vi "Version_2.0_Single_Column_Code.vi"() -> ()   [LabVIEW 2020] (continued)
                        n8405 = local write "Reminder of the \nVolume to be \nPumped"(w8823) -> ()
                      }
                      frame #1 {
                        n8406 = stacked-sequence {
                          frame #0 {
                            # "Switch to Port-4"
                            # "Port-4 of pump is connected to Buffer-A"
                            n8407 = local read "VISA Refnum in\nfor Pump"() -> (w8907:refnum<visa-resource-name>)
                            n8408 = local read "Port for \nA2-Wash"() -> (w8906:string)
                            n8409 = call "PortChanger (SubVI).vi"("Port Number"=w8906, "VISA Refnum in"=w8907) -> ()  [unwired: 10 in]
                          }
                          frame #1 {
                            n8410 = local read "VISA Refnum in\nfor Pump"() -> (w8908:refnum<visa-resource-name>)
                            n8411 = call "ProcessCompletionWaiter (SubVI).vi"("VISA Refnum in"=w8908) -> ()  [unwired: 11 in]
                          }
                          frame #2 {
                            n8412 = local read "Buffer-A2 PickUp \nFlow Rate (ul/min)"() -> (w8911:dbl)
                            n8413 = local read "Buffer-A2 Pumping\nResolution"() -> (w8910:T2)
                            n8414 = local read "VISA Refnum in\nfor Pump"() -> (w8913:refnum<visa-resource-name>)
                            n8415 = local read "Reminder of the \nVolume to be \nPumped"() -> (w8909:dbl)
                            n8416 = local read "Volume of Syringe"() -> (w8912:dbl)
                            n8417 = call "RPickUp(SubVI).vi"("Volume to be picked up"=w8909, "Volume of Syringe"=w8912, "Resolution of PickUP"=w8910, "PickUp Flow Rate (ul/min)"=w8911, "VISA Refnum in"=w8913) -> ()  [unwired: 6 in, 1 out]
                          }
                          frame #3 {
                            n8418 = local read "Stopper that ends \nthe main loops"() -> (w8914:bool)
                            n8419 = local read "VISA Refnum in\nfor Pump"() -> (w8915:refnum<visa-resource-name>)
                            n8420 = case shown="True" w8914 {
                              frame False {
                              }
                              frame True {
                                n8421 = local read "VISA Refnum in\nfor Pump"() -> (w8916:refnum<visa-resource-name>)
                                n8422 = call "HardStopCurrentProcess (SubVI).vi"("VISA Refnum in"=w8916) -> ()  [unwired: 11 in]
                              }
                            }
                            n8423 = call "ProcessCompletionWaiter (SubVI).vi"("VISA Refnum in"=w8915) -> ()  [unwired: 11 in]
                          }
                          frame #4 {
                            # "Reads the initial Plunger Position for computing the volume dispensed"
                            n8424 = local read "VISA Refnum in\nfor Pump"() -> (w8918:refnum<visa-resource-name>)
                            n8425 = call "AbsolutePlungerPosition (SubVI).vi"("VISA Refnum in"=w8918) -> ("Plunger Position"=w8917:i32)  [unwired: 10 in]
                            n8426 = local write "Initial Plunger Position"(w8917) -> ()
                          }
                          frame #5 {
                            # "Switch to Port-2"
                            # "Port-2 of the pump is conncted to column-1 of chip"
                            n8427 = local read "VISA Refnum in\nfor Pump"() -> (w8920:refnum<visa-resource-name>)
                            n8428 = call "PortChanger (SubVI).vi"("Port Number"="2", "VISA Refnum in"=w8920) -> ()  [unwired: 10 in]
                          }
                          frame #6 {
                            n8429 = local read "Stopper that ends \nthe main loops"() -> (w8921:bool)
                            n8430 = local read "VISA Refnum in\nfor Pump"() -> (w8922:refnum<visa-resource-name>)
                            n8431 = case shown="True" w8921 {
                              frame False {
                              }
                              frame True {
                                n8432 = local read "VISA Refnum in\nfor Pump"() -> (w8923:refnum<visa-resource-name>)
                                n8433 = call "HardStopCurrentProcess (SubVI).vi"("VISA Refnum in"=w8923) -> ()  [unwired: 11 in]
                              }
                            }
                            n8434 = call "ProcessCompletionWaiter (SubVI).vi"("VISA Refnum in"=w8922) -> ()  [unwired: 11 in]
                          }
                          frame #7 {
                            # "Keeps the AMF valve after column-1 open and valve after column-2 closed"
                            n8435 = local read "Buffer-A2 Dispense\nFlow Rate (ul/min)"() -> (w8936:dbl)
                            n8436 = local read "Buffer-A2 Pumping\nResolution"() -> (w8935:T2)
                            n8437 = local read "VISA Refnum in\nfor Pump"() -> (w8938:refnum<visa-resource-name>)
                            n8438 = local write "Pause Data Collection"(FALSE ("Pause Data Collection")) -> ()
                            n8439 = local write "Valve V3 Open"(TRUE ("Valve V3 Open")) -> ()
                            n8440 = local write "Valve V4 Open"(TRUE ("Valve V4 Open")) -> ()
                            n8441 = local write "Valve V1 Open"(TRUE ("Valve V1 Open")) -> ()
                            n8442 = local write "Valve V2 Open"(FALSE ("Valve V2 Open")) -> ()
                            n8443 = local read "Volume of Syringe"() -> (w8937:dbl)
                            n8444 = call "GoToAbsolutePosition(SubVI).vi"("Absolute Volume Position in Syringe (in ul)"=0.0 ("Volume to be Dispensed"), "Volume of Syringe"=w8937, "Resolution of Pumping"=w8935, "Flow Rate (ul/min)"=w8936, "VISA Refnum in"=w8938) -> ()  [unwired: 6 in, 1 out]
                            n8445 = local write "External Valve \nOpen"(FALSE ("External Valve \nOpen")) -> ()
                            n8446 = local write "Valve V5 Open"(TRUE ("Valve V5 Open")) -> ()
                            n8447 = local write "Valve V8 Open"(TRUE ("Valve V8 Open")) -> ()
                            n8448 = local write "Valve V6 Open"(TRUE ("Valve V6 Open")) -> ()
                            n8449 = local write "Valve V7 Open"(TRUE ("Valve V7 Open")) -> ()
                          }
                          frame #8 {
                            n8450 = local read "Initial Plunger Position"() -> (w8941:dbl)
                            n8451 = local read "Buffer-A2 Pumping\nResolution"() -> (w8940:T2)
                            n8452 = local read "VISA Refnum in\nfor Pump"() -> (w8942:refnum<visa-resource-name>)
                            n8453 = local read "Volume of Syringe"() -> (w8939:dbl)
                            n8454 = while {
                              tunnel: w8941 -> [w8948]
                              tunnel: w8942 -> [w8947]
                              tunnel: w8940 -> [w8946]
                              tunnel: w8939 -> [w8945]
                              stop <- w8943 stop-if-true
                              n8455 = Wait (ms)(milliseconds to wait=u32 100) -> ()  [unwired: 1 out]
                              n8456 = stacked-sequence {
                                tunnel: w8948 -> [w8954 _]
                                tunnel: w8947 -> [w8953 w8974]
                                tunnel: w8946 -> [w8952 _]
                                tunnel: w8945 -> [w8951 _]
                                tunnel: [_ w8971] -> w8943
                                frame #0 {
                                n8457 = call "AbsolutePlungerPosition (SubVI).vi"("VISA Refnum in"=w8953) -> ("Plunger Position"=w8950:i32)  [unwired: 10 in]
                                n8458 = case shown="\"Standard Pumping\", Default" w8952 {
                                tunnel: w8954 -> [w8959 w8968]
                                tunnel: w8950 -> [w8960 w8967]
                                tunnel: [w8958 w8965] -> w8949
                                tunnel: w8951 -> [w8957 w8966]
                                frame "Standard Pumping", Default {
                                n8459 = Subtract(x=w8959, y=w8960) -> (x-y=w8956:dbl)
                                n8460 = Absolute Value(x=w8956) -> (abs(x)=w8955:dbl)
                                n8461 = Multiply(x=w8955, y=w8957) -> (x*y=w8962:dbl)
                                n8462 = Divide(x=w8962, y=3000.0) -> (x/y=w8958:dbl)
                                }
                                frame "High Resolution Pumping" {
                                n8463 = Subtract(x=w8968, y=w8967) -> (x-y=w8964:dbl)
                                n8464 = Absolute Value(x=w8964) -> (abs(x)=w8963:dbl)
                                n8465 = Multiply(x=w8963, y=w8966) -> (x*y=w8970:dbl)
                                n8466 = Divide(x=w8970, y=24000.0) -> (x/y=w8965:dbl)
                                }
                                }
                                n8467 = local write "Volume being Injected \nin this process"(w8949) -> ()
                                }
                                frame #1 {
                                n8468 = local read "Stop for End of \nExperiment \nand Data Writing"() -> (w8973:bool)
                                n8469 = call "LSPOneStatus (SubVI).vi"("VISA Refnum in"=w8974) -> ("read buffer"=w8976:string)  [unwired: 10 in]
                                n8470 = call <vilib>:"Trim Whitespace.vi"("string"=w8976) -> ("trimmed string"=w8975:string)  [unwired: 1 in]
                                n8471 = Equal?(x=w8975, y="/0`\u0003") -> (x = y?=w8972:bool)
                                n8472 = Or(x=w8972, y=w8973) -> (x .or. y?=w8971:bool)
                                }
                              }
                            }
                          }
                          frame #9 {
                            n8473 = local read "Stop for End of \nExperiment \nand Data Writing"() -> (w8978:bool)
                            n8474 = local write "Pause Data Collection"(TRUE ("Pause Data Collection")) -> ()
                            n8475 = local write "Valve V2 Open"(FALSE ("Valve V2 Open")) -> ()
                            n8476 = local write "Start the Process"(FALSE) -> ()
                            n8477 = local write "Valve V1 Open"(FALSE ("Valve V1 Open")) -> ()
                            n8478 = case shown="True" w8978 {
                              frame False {
                              }
                              frame True {
                                n8479 = local read "VISA Refnum in\nfor Pump"() -> (w8984:refnum<visa-resource-name>)
                                n8480 = call "HardStopCurrentProcess (SubVI).vi"("VISA Refnum in"=w8984) -> ()  [unwired: 11 in]
                              }
                            }
                            n8481 = Wait (ms)(milliseconds to wait=u32 500) -> ()  [unwired: 1 out]
                          }
                          frame #10 {
                            n8482 = local write "Volume being Injected \nin this process"(0.0 ("Volume being Injected \nin this process")) -> ()
                          }
                        }
                      }
                    }
                  }
                }
              }
              frame True {
                n8483 = local write "Pause Data Collection"(FALSE ("Pause Data Collection")) -> ()
              }
            }
          }
          frame "Inject Buffer B, Column 1 with 4 SOD Valves" {
            n8484 = local read "Stopper that ends \nthe main loops"() -> (w8987:bool)
            n8485 = case shown="False" w8987 {
              frame False {
                n8486 = local read "Start the Process"() -> (w8988:bool)
                n8487 = case shown="True" w8988 {
                  frame False {
                    n8488 = local read "Stopper that ends \nthe main loops"() -> (w8990:bool)
                    n8489 = local read "Start the Process"() -> (w8989:bool)
                    n8490 = Or(x=w8990, y=w8989) -> (x .or. y?=w8991:bool)
                    n8491 = case shown="False" w8991 {
                      frame False {
                        n8492 = while {
                          stop <- w8994 stop-if-true
                          n8493 = local read "Stop for End of \nExperiment \nand Data Writing"() -> (w8993:bool)
                          n8494 = local read "Stopper that ends \nthe main loops"() -> (w8996:bool)
                          n8495 = local read "Start the Process"() -> (w8995:bool)
                          n8496 = Wait (ms)(milliseconds to wait=u32 10) -> ()  [unwired: 1 out]
                          n8497 = Or(x=w8996, y=w8995) -> (x .or. y?=w8994:bool)
                          n8498 = local write "Stopper that ends \nthe main loops"(w8993) -> ()
                        }
                        n8499 = One Button Dialog(message="Please Select the Process and Press 'Start the Process' Button") -> ()  [unwired: 1 in, 1 out]
                      }
                      frame True {
                      }
                    }
                  }
                  frame True {
                    n8500 = stacked-sequence {
                      frame #0 {
                        n8501 = local read "Apparent Volume\nof Syringe"() -> (w9000:dbl)
                        n8502 = local read "Buffer-B Volume \nto be  Pumped"() -> (w9001:dbl)
                        n8503 = Quotient & Remainder(x=w9001, y=w9000) -> (x-y*floor(x/y)=w8998:dbl, floor(x/y)=w8999:dbl)
                        n8504 = for {
                          N: w8999 -> [_]
                          n8505 = stacked-sequence {
                            frame #0 {
                              # "Switch to Port-7"
                              # "Port-7 of pump is connected to Buffer-B"
                              n8506 = local read "VISA Refnum in\nfor Pump"() -> (w9003:refnum<visa-resource-name>)
                              n8507 = local read "Port for \nB-Elution"() -> (w9002:string)
                              n8508 = call "PortChanger (SubVI).vi"("Port Number"=w9002, "VISA Refnum in"=w9003) -> ()  [unwired: 10 in]
                            }
                            frame #1 {
                              n8509 = local read "VISA Refnum in\nfor Pump"() -> (w9004:refnum<visa-resource-name>)
                              n8510 = call "ProcessCompletionWaiter (SubVI).vi"("VISA Refnum in"=w9004) -> ()  [unwired: 11 in]
                            }
                            frame #2 {
                              n8511 = local read "Buffer-B PickUp \nFlow Rate (ul/min)"() -> (w9007:dbl)
                              n8512 = local read "Buffer-B Pumping\nResolution"() -> (w9006:T2)
                              n8513 = local read "VISA Refnum in\nfor Pump"() -> (w9009:refnum<visa-resource-name>)
                              n8514 = local read "Apparent Volume\nof Syringe"() -> (w9005:dbl)
                              n8515 = local read "Volume of Syringe"() -> (w9008:dbl)
                              n8516 = call "RPickUp(SubVI).vi"("Volume to be picked up"=w9005, "Volume of Syringe"=w9008, "Resolution of PickUP"=w9006, "PickUp Flow Rate (ul/min)"=w9007, "VISA Refnum in"=w9009) -> ()  [unwired: 6 in, 1 out]
                            }
                            frame #3 {
                              n8517 = local read "Stopper that ends \nthe main loops"() -> (w9010:bool)
                              n8518 = local read "VISA Refnum in\nfor Pump"() -> (w9011:refnum<visa-resource-name>)
                              n8519 = case shown="True" w9010 {
                                frame False {
                                }
                                frame True {
                                n8520 = local read "VISA Refnum in\nfor Pump"() -> (w9012:refnum<visa-resource-name>)
                                n8521 = call "HardStopCurrentProcess (SubVI).vi"("VISA Refnum in"=w9012) -> ()  [unwired: 11 in]
                                }
                              }
                              n8522 = call "ProcessCompletionWaiter (SubVI).vi"("VISA Refnum in"=w9011) -> ()  [unwired: 11 in]
                            }
                            frame #4 {
                              # "Reads the initial Plunger Position for computing the volume dispensed"
                              n8523 = local read "VISA Refnum in\nfor Pump"() -> (w9014:refnum<visa-resource-name>)
                              n8524 = call "AbsolutePlungerPosition (SubVI).vi"("VISA Refnum in"=w9014) -> ("Plunger Position"=w9013:i32)  [unwired: 10 in]
                              n8525 = local write "Initial Plunger Position"(w9013) -> ()
                            }
                            frame #5 {
                              # "Switch to Port-8"
                              # "Port-8 of the pump is conncted to column-1 of chip"
                              n8526 = local read "VISA Refnum in\nfor Pump"() -> (w9016:refnum<visa-resource-name>)
                              n8527 = call "PortChanger (SubVI).vi"("Port Number"="8", "VISA Refnum in"=w9016) -> ()  [unwired: 10 in]
                            }
                            frame #6 {
                              n8528 = local read "Stopper that ends \nthe main loops"() -> (w9017:bool)
                              n8529 = local read "VISA Refnum in\nfor Pump"() -> (w9018:refnum<visa-resource-name>)
                              n8530 = case shown="True" w9017 {
                                frame False {
                                }
                                frame True {
                                n8531 = local read "VISA Refnum in\nfor Pump"() -> (w9019:refnum<visa-resource-name>)
                                n8532 = call "HardStopCurrentProcess (SubVI).vi"("VISA Refnum in"=w9019) -> ()  [unwired: 11 in]
                                }
                              }
                              n8533 = call "ProcessCompletionWaiter (SubVI).vi"("VISA Refnum in"=w9018) -> ()  [unwired: 11 in]
                            }
                            frame #7 {
                              # "Keeps the AMF valve after column-1 open and valve after column-2 closed"
                              n8534 = local read "Buffer-B Dispense\nFlow Rate (ul/min)"() -> (w9032:dbl)
                              n8535 = local read "Buffer-B Pumping\nResolution"() -> (w9031:T2)
                              n8536 = local read "VISA Refnum in\nfor Pump"() -> (w9034:refnum<visa-resource-name>)
                              n8537 = local write "Pause Data Collection"(FALSE ("Pause Data Collection")) -> ()
                              n8538 = local write "Valve V1 Open"(TRUE ("Valve V1 Open")) -> ()
                              n8539 = local write "Valve V3 Open"(FALSE ("Valve V3 Open")) -> ()
                              n8540 = local write "Valve V2 Open"(TRUE ("Valve V2 Open")) -> ()
                              n8541 = local write "Valve V4 Open"(FALSE ("Valve V4 Open")) -> ()
                              n8542 = local read "Volume of Syringe"() -> (w9033:dbl)
                              n8543 = call "GoToAbsolutePosition(SubVI).vi"("Absolute Volume Position in Syringe (in ul)"=0.0 ("Volume to be Dispensed"), "Volume of Syringe"=w9033, "Resolution of Pumping"=w9031, "Flow Rate (ul/min)"=w9032, "VISA Refnum in"=w9034) -> ()  [unwired: 6 in, 1 out]
                              n8544 = local write "External Valve \nOpen"(TRUE ("External Valve \nOpen")) -> ()
                              n8545 = local write "Valve V8 Open"(FALSE ("Valve V8 Open")) -> ()
                              n8546 = local write "Valve V6 Open"(FALSE ("Valve V6 Open")) -> ()
                              n8547 = local write "Valve V7 Open"(FALSE ("Valve V7 Open")) -> ()
                              n8548 = local write "Valve V5 Open"(FALSE ("Valve V5 Open")) -> ()
                            }
                            frame #8 {
                              n8549 = local read "Initial Plunger Position"() -> (w9037:dbl)
                              n8550 = local read "Buffer-B Pumping\nResolution"() -> (w9036:T2)
                              n8551 = local read "VISA Refnum in\nfor Pump"() -> (w9038:refnum<visa-resource-name>)
                              n8552 = local read "Volume of Syringe"() -> (w9035:dbl)
                              n8553 = while {
                                tunnel: w9037 -> [w9044]
                                tunnel: w9038 -> [w9043]
                                tunnel: w9036 -> [w9042]
                                tunnel: w9035 -> [w9041]
                                stop <- w9039 stop-if-true
                                n8554 = Wait (ms)(milliseconds to wait=u32 100) -> ()  [unwired: 1 out]
                                n8555 = stacked-sequence {
                                tunnel: w9044 -> [w9050 _]
                                tunnel: w9043 -> [w9049 w9070]
                                tunnel: w9042 -> [w9048 _]
                                tunnel: w9041 -> [w9047 _]
                                tunnel: [_ w9067] -> w9039
                                frame #0 {
                                n8556 = call "AbsolutePlungerPosition (SubVI).vi"("VISA Refnum in"=w9049) -> ("Plunger Position"=w9046:i32)  [unwired: 10 in]
                                n8557 = case shown="\"Standard Pumping\", Default" w9048 {
                                tunnel: w9050 -> [w9055 w9064]
                                tunnel: w9046 -> [w9056 w9063]
                                tunnel: [w9054 w9061] -> w9045
                                tunnel: w9047 -> [w9053 w9062]
                                frame "Standard Pumping", Default {
                                n8558 = Subtract(x=w9055, y=w9056) -> (x-y=w9052:dbl)
                                n8559 = Absolute Value(x=w9052) -> (abs(x)=w9051:dbl)
                                n8560 = Multiply(x=w9051, y=w9053) -> (x*y=w9058:dbl)
                                n8561 = Divide(x=w9058, y=3000.0) -> (x/y=w9054:dbl)
                                }
                                frame "High Resolution Pumping" {
                                n8562 = Subtract(x=w9064, y=w9063) -> (x-y=w9060:dbl)
                                n8563 = Absolute Value(x=w9060) -> (abs(x)=w9059:dbl)
                                n8564 = Multiply(x=w9059, y=w9062) -> (x*y=w9066:dbl)
                                n8565 = Divide(x=w9066, y=24000.0) -> (x/y=w9061:dbl)
                                }
                                }
                                n8566 = local write "Volume being Injected \nin this process"(w9045) -> ()
                                }
                                frame #1 {
                                n8567 = call "LSPOneStatus (SubVI).vi"("VISA Refnum in"=w9070) -> ("read buffer"=w9072:string)  [unwired: 10 in]
                                n8568 = local read "Stopper that ends \nthe main loops"() -> (w9069:bool)
                                n8569 = call <vilib>:"Trim Whitespace.vi"("string"=w9072) -> ("trimmed string"=w9071:string)  [unwired: 1 in]
                                n8570 = Equal?(x=w9071, y="/0`\u0003") -> (x = y?=w9068:bool)
                                n8571 = Or(x=w9068, y=w9069) -> (x .or. y?=w9067:bool)
                                }
                                }
                              }
                            }
                            frame #9 {
                              n8572 = local read "Stopper that ends \nthe main loops"() -> (w9074:bool)
                              n8573 = local write "Pause Data Collection"(TRUE ("Pause Data Collection")) -> ()
                              n8574 = local write "Valve V2 Open"(FALSE ("Valve V2 Open")) -> ()
                              n8575 = local write "Valve V4 Open"(FALSE ("Valve V4 Open")) -> ()
                              n8576 = Wait (ms)(milliseconds to wait=u32 500) -> ()  [unwired: 1 out]
                              n8577 = local write "Valve V1 Open"(FALSE ("Valve V1 Open")) -> ()
                              n8578 = local write "Valve V3 Open"(FALSE ("Valve V3 Open")) -> ()
                              n8579 = case shown="True" w9074 {
                                frame False {
                                }
                                frame True {
                                n8580 = local read "VISA Refnum in\nfor Pump"() -> (w9084:refnum<visa-resource-name>)
                                n8581 = call "HardStopCurrentProcess (SubVI).vi"("VISA Refnum in"=w9084) -> ()  [unwired: 11 in]
                                }
                              }
                              n8582 = local write "Valve V5 Open"(FALSE ("Valve V5 Open")) -> ()
                              n8583 = local write "Valve V6 Open"(FALSE ("Valve V6 Open")) -> ()
                              n8584 = local write "Valve V7 Open"(FALSE ("Valve V7 Open")) -> ()
                            }
                            frame #10 {
                              n8585 = local write "Volume being Injected \nin this process"(0.0 ("Volume being Injected \nin this process")) -> ()
                            }
                          }
                        }
                        n8586 = local write "Reminder of the \nVolume to be \nPumped"(w8998) -> ()
                      }
                      frame #1 {
                        n8587 = stacked-sequence {
                          frame #0 {
                            # "Switch to Port-7"
                            # "Port-7 of pump is connected to Buffer-B"
                            n8588 = local read "VISA Refnum in\nfor Pump"() -> (w9087:refnum<visa-resource-name>)
                            n8589 = local read "Port for \nB-Elution"() -> (w9086:string)
                            n8590 = call "PortChanger (SubVI).vi"("Port Number"=w9086, "VISA Refnum in"=w9087) -> ()  [unwired: 10 in]
                          }
                          frame #1 {
                            n8591 = local read "VISA Refnum in\nfor Pump"() -> (w9088:refnum<visa-resource-name>)
                            n8592 = call "ProcessCompletionWaiter (SubVI).vi"("VISA Refnum in"=w9088) -> ()  [unwired: 11 in]
                          }
                          frame #2 {
                            n8593 = local read "Buffer-B PickUp \nFlow Rate (ul/min)"() -> (w9091:dbl)
                            n8594 = local read "Buffer-B Pumping\nResolution"() -> (w9090:T2)
                            n8595 = local read "VISA Refnum in\nfor Pump"() -> (w9093:refnum<visa-resource-name>)
                            n8596 = local read "Reminder of the \nVolume to be \nPumped"() -> (w9089:dbl)
                            n8597 = local read "Volume of Syringe"() -> (w9092:dbl)
                            n8598 = call "RPickUp(SubVI).vi"("Volume to be picked up"=w9089, "Volume of Syringe"=w9092, "Resolution of PickUP"=w9090, "PickUp Flow Rate (ul/min)"=w9091, "VISA Refnum in"=w9093) -> ()  [unwired: 6 in, 1 out]
                          }
                          frame #3 {
                            n8599 = local read "Stopper that ends \nthe main loops"() -> (w9094:bool)
                            n8600 = local read "VISA Refnum in\nfor Pump"() -> (w9095:refnum<visa-resource-name>)
                            n8601 = case shown="True" w9094 {
                              frame False {
                              }
                              frame True {
                                n8602 = local read "VISA Refnum in\nfor Pump"() -> (w9096:refnum<visa-resource-name>)
                                n8603 = call "HardStopCurrentProcess (SubVI).vi"("VISA Refnum in"=w9096) -> ()  [unwired: 11 in]
                              }
                            }
                            n8604 = call "ProcessCompletionWaiter (SubVI).vi"("VISA Refnum in"=w9095) -> ()  [unwired: 11 in]
                          }
                          frame #4 {
                            # "Reads the initial Plunger Position for computing the volume dispensed"
                            n8605 = local read "VISA Refnum in\nfor Pump"() -> (w9098:refnum<visa-resource-name>)
                            n8606 = call "AbsolutePlungerPosition (SubVI).vi"("VISA Refnum in"=w9098) -> ("Plunger Position"=w9097:i32)  [unwired: 10 in]
                            n8607 = local write "Initial Plunger Position"(w9097) -> ()
                          }
                          frame #5 {
                            # "Switch to Port-2"
                            # "Port-2 of the pump is conncted to column-1 of chip"
                            n8608 = local read "VISA Refnum in\nfor Pump"() -> (w9100:refnum<visa-resource-name>)
                            n8609 = call "PortChanger (SubVI).vi"("Port Number"="8", "VISA Refnum in"=w9100) -> ()  [unwired: 10 in]
                          }
                          frame #6 {
                            n8610 = local read "Stopper that ends \nthe main loops"() -> (w9101:bool)
                            n8611 = local read "VISA Refnum in\nfor Pump"() -> (w9102:refnum<visa-resource-name>)
                            n8612 = case shown="True" w9101 {
                              frame False {
                              }
                              frame True {
                                n8613 = local read "VISA Refnum in\nfor Pump"() -> (w9103:refnum<visa-resource-name>)
                                n8614 = call "HardStopCurrentProcess (SubVI).vi"("VISA Refnum in"=w9103) -> ()  [unwired: 11 in]
                              }
                            }
                            n8615 = call "ProcessCompletionWaiter (SubVI).vi"("VISA Refnum in"=w9102) -> ()  [unwired: 11 in]
                          }
                          frame #7 {
                            # "Keeps the AMF valve after column-1 open and valve after column-2 closed"
                            n8616 = local read "Buffer-B Dispense\nFlow Rate (ul/min)"() -> (w9116:dbl)
                            n8617 = local read "Buffer-B Pumping\nResolution"() -> (w9115:T2)
                            n8618 = local read "VISA Refnum in\nfor Pump"() -> (w9118:refnum<visa-resource-name>)
                            n8619 = local write "Pause Data Collection"(FALSE ("Pause Data Collection")) -> ()
                            n8620 = local write "Valve V1 Open"(TRUE ("Valve V1 Open")) -> ()
                            n8621 = local write "Valve V3 Open"(FALSE ("Valve V3 Open")) -> ()
                            n8622 = local write "Valve V2 Open"(TRUE ("Valve V2 Open")) -> ()
                            n8623 = local write "Valve V4 Open"(FALSE ("Valve V4 Open")) -> ()
                            n8624 = local read "Volume of Syringe"() -> (w9117:dbl)
                            n8625 = call "GoToAbsolutePosition(SubVI).vi"("Absolute Volume Position in Syringe (in ul)"=0.0 ("Volume to be Dispensed"), "Volume of Syringe"=w9117, "Resolution of Pumping"=w9115, "Flow Rate (ul/min)"=w9116, "VISA Refnum in"=w9118) -> ()  [unwired: 6 in, 1 out]
                            n8626 = local write "External Valve \nOpen"(TRUE ("External Valve \nOpen")) -> ()
                            n8627 = local write "Valve V8 Open"(FALSE ("Valve V8 Open")) -> ()
                            n8628 = local write "Valve V6 Open"(FALSE ("Valve V6 Open")) -> ()
                            n8629 = local write "Valve V7 Open"(FALSE ("Valve V7 Open")) -> ()
                            n8630 = local write "Valve V5 Open"(FALSE ("Valve V5 Open")) -> ()
                          }
                          frame #8 {
                            n8631 = local read "Initial Plunger Position"() -> (w9121:dbl)
                            n8632 = local read "Buffer-B Pumping\nResolution"() -> (w9120:T2)
                            n8633 = local read "VISA Refnum in\nfor Pump"() -> (w9122:refnum<visa-resource-name>)
                            n8634 = local read "Volume of Syringe"() -> (w9119:dbl)
                            n8635 = while {
                              tunnel: w9121 -> [w9128]
                              tunnel: w9122 -> [w9127]
                              tunnel: w9120 -> [w9126]
                              tunnel: w9119 -> [w9125]
                              stop <- w9123 stop-if-true
                              n8636 = Wait (ms)(milliseconds to wait=u32 100) -> ()  [unwired: 1 out]
                              n8637 = stacked-sequence {
                                tunnel: w9128 -> [w9134 _]
                                tunnel: w9127 -> [w9133 w9154]
                                tunnel: w9126 -> [w9132 _]
                                tunnel: w9125 -> [w9131 _]
                                tunnel: [_ w9151] -> w9123
                                frame #0 {
                                n8638 = call "AbsolutePlungerPosition (SubVI).vi"("VISA Refnum in"=w9133) -> ("Plunger Position"=w9130:i32)  [unwired: 10 in]
                                n8639 = case shown="\"Standard Pumping\", Default" w9132 {
                                tunnel: w9134 -> [w9139 w9148]
                                tunnel: w9130 -> [w9140 w9147]
                                tunnel: [w9138 w9145] -> w9129
                                tunnel: w9131 -> [w9137 w9146]
                                frame "Standard Pumping", Default {
                                n8640 = Subtract(x=w9139, y=w9140) -> (x-y=w9136:dbl)
                                n8641 = Absolute Value(x=w9136) -> (abs(x)=w9135:dbl)
                                n8642 = Multiply(x=w9135, y=w9137) -> (x*y=w9142:dbl)
                                n8643 = Divide(x=w9142, y=3000.0) -> (x/y=w9138:dbl)
                                }
                                frame "High Resolution Pumping" {
                                n8644 = Subtract(x=w9148, y=w9147) -> (x-y=w9144:dbl)
                                n8645 = Absolute Value(x=w9144) -> (abs(x)=w9143:dbl)
                                n8646 = Multiply(x=w9143, y=w9146) -> (x*y=w9150:dbl)
                                n8647 = Divide(x=w9150, y=24000.0) -> (x/y=w9145:dbl)
                                }
                                }
                                n8648 = local write "Volume being Injected \nin this process"(w9129) -> ()
                                }
                                frame #1 {
                                n8649 = call "LSPOneStatus (SubVI).vi"("VISA Refnum in"=w9154) -> ("read buffer"=w9156:string)  [unwired: 10 in]
                                n8650 = local read "Stopper that ends \nthe main loops"() -> (w9153:bool)
                                n8651 = call <vilib>:"Trim Whitespace.vi"("string"=w9156) -> ("trimmed string"=w9155:string)  [unwired: 1 in]
                                n8652 = Equal?(x=w9155, y="/0`\u0003") -> (x = y?=w9152:bool)
                                n8653 = Or(x=w9152, y=w9153) -> (x .or. y?=w9151:bool)
                                }
                              }
                            }
                          }
                          frame #9 {
                            n8654 = local read "Stopper that ends \nthe main loops"() -> (w9158:bool)
                            n8655 = local write "Pause Data Collection"(TRUE ("Pause Data Collection")) -> ()
                            n8656 = local write "Valve V2 Open"(FALSE ("Valve V2 Open")) -> ()
                            n8657 = local write "Start the Process"(FALSE) -> ()
                            n8658 = local write "Valve V4 Open"(FALSE ("Valve V4 Open")) -> ()
                            n8659 = Wait (ms)(milliseconds to wait=u32 500) -> ()  [unwired: 1 out]
                            n8660 = local write "Valve V1 Open"(FALSE ("Valve V1 Open")) -> ()
                            n8661 = local write "Valve V3 Open"(FALSE ("Valve V3 Open")) -> ()
                            n8662 = case shown="True" w9158 {
                              frame False {
                              }
                              frame True {
                                n8663 = local read "VISA Refnum in\nfor Pump"() -> (w9169:refnum<visa-resource-name>)
                                n8664 = call "HardStopCurrentProcess (SubVI).vi"("VISA Refnum in"=w9169) -> ()  [unwired: 11 in]
                              }
                            }
                            n8665 = local write "Valve V5 Open"(FALSE ("Valve V5 Open")) -> ()
                            n8666 = local write "Valve V6 Open"(FALSE ("Valve V6 Open")) -> ()
                            n8667 = local write "Valve V7 Open"(FALSE ("Valve V7 Open")) -> ()
                          }
                          frame #10 {
                            n8668 = local write "Volume being Injected \nin this process"(0.0 ("Volume being Injected \nin this process")) -> ()
                          }
                        }
                      }
                    }
                  }
                }
              }
              frame True {
                n8669 = local write "Pause Data Collection"(FALSE ("Pause Data Collection")) -> ()
              }
            }
          }
          frame "Single Column Elution Buffer-B" {
            n8670 = local read "Stopper that ends \nthe main loops"() -> (w9172:bool)
            n8671 = case shown="False" w9172 {
              frame False {
                n8672 = local read "Start the Process"() -> (w9173:bool)
                n8673 = case shown="True" w9173 {
                  frame False {
                    n8674 = local read "Stopper that ends \nthe main loops"() -> (w9175:bool)
                    n8675 = local read "Start the Process"() -> (w9174:bool)
                    n8676 = Or(x=w9175, y=w9174) -> (x .or. y?=w9176:bool)
                    n8677 = case shown="False" w9176 {
                      frame False {
                        n8678 = while {
                          stop <- w9179 stop-if-true
                          n8679 = local read "Stop for End of \nExperiment \nand Data Writing"() -> (w9178:bool)
                          n8680 = local read "Stopper that ends \nthe main loops"() -> (w9181:bool)
                          n8681 = local read "Start the Process"() -> (w9180:bool)
                          n8682 = Wait (ms)(milliseconds to wait=u32 10) -> ()  [unwired: 1 out]
                          n8683 = Or(x=w9181, y=w9180) -> (x .or. y?=w9179:bool)
                          n8684 = local write "Stopper that ends \nthe main loops"(w9178) -> ()
                        }
                        n8685 = One Button Dialog(message="Please Select the Process and Press 'Start the Process' Button") -> ()  [unwired: 1 in, 1 out]
                      }
                      frame True {
                      }
                    }
                  }
                  frame True {
                    n8686 = stacked-sequence {
                      frame #0 {
                        n8687 = local read "Apparent Volume\nof Syringe"() -> (w9185:dbl)
                        n8688 = local read "Buffer-B Volume \nto be  Pumped"() -> (w9186:dbl)
                        n8689 = Quotient & Remainder(x=w9186, y=w9185) -> (x-y*floor(x/y)=w9183:dbl, floor(x/y)=w9184:dbl)
                        n8690 = for {
                          N: w9184 -> [_]
                          n8691 = stacked-sequence {
                            frame #0 {
                              # "Switch to Port-7"
                              # "Port-7 of pump is connected to Buffer-B"
                              n8692 = local read "VISA Refnum in\nfor Pump"() -> (w9188:refnum<visa-resource-name>)
                              n8693 = local read "Port for \nB-Elution"() -> (w9187:string)
                              n8694 = call "PortChanger (SubVI).vi"("Port Number"=w9187, "VISA Refnum in"=w9188) -> ()  [unwired: 10 in]
                            }
                            frame #1 {
                              n8695 = local read "VISA Refnum in\nfor Pump"() -> (w9189:refnum<visa-resource-name>)
                              n8696 = call "ProcessCompletionWaiter (SubVI).vi"("VISA Refnum in"=w9189) -> ()  [unwired: 11 in]
                            }
                            frame #2 {
                              n8697 = local read "Buffer-B PickUp \nFlow Rate (ul/min)"() -> (w9192:dbl)
                              n8698 = local read "Buffer-B Pumping\nResolution"() -> (w9191:T2)
                              n8699 = local read "VISA Refnum in\nfor Pump"() -> (w9194:refnum<visa-resource-name>)
                              n8700 = local read "Apparent Volume\nof Syringe"() -> (w9190:dbl)
                              n8701 = local read "Volume of Syringe"() -> (w9193:dbl)
                              n8702 = call "RPickUp(SubVI).vi"("Volume to be picked up"=w9190, "Volume of Syringe"=w9193, "Resolution of PickUP"=w9191, "PickUp Flow Rate (ul/min)"=w9192, "VISA Refnum in"=w9194) -> ()  [unwired: 6 in, 1 out]
                            }
                            frame #3 {
                              n8703 = local read "Stopper that ends \nthe main loops"() -> (w9195:bool)
                              n8704 = local read "VISA Refnum in\nfor Pump"() -> (w9196:refnum<visa-resource-name>)
                              n8705 = case shown="True" w9195 {
                                frame False {
                                }
                                frame True {
                                n8706 = local read "VISA Refnum in\nfor Pump"() -> (w9197:refnum<visa-resource-name>)
                                n8707 = call "HardStopCurrentProcess (SubVI).vi"("VISA Refnum in"=w9197) -> ()  [unwired: 11 in]
                                }
                              }
                              n8708 = call "ProcessCompletionWaiter (SubVI).vi"("VISA Refnum in"=w9196) -> ()  [unwired: 11 in]
                            }
                            frame #4 {
                              # "Reads the initial Plunger Position for computing the volume dispensed"
                              n8709 = local read "VISA Refnum in\nfor Pump"() -> (w9199:refnum<visa-resource-name>)
                              n8710 = call "AbsolutePlungerPosition (SubVI).vi"("VISA Refnum in"=w9199) -> ("Plunger Position"=w9198:i32)  [unwired: 10 in]
                              n8711 = local write "Initial Plunger Position"(w9198) -> ()
                            }
                            frame #5 {
                              # "Switch to Port-8"
                              # "Port-8 of the pump is conncted to column-1 of chip"
                              n8712 = local read "VISA Refnum in\nfor Pump"() -> (w9201:refnum<visa-resource-name>)
                              n8713 = call "PortChanger (SubVI).vi"("Port Number"="8", "VISA Refnum in"=w9201) -> ()  [unwired: 10 in]
                            }
                            frame #6 {
                              n8714 = local read "Stopper that ends \nthe main loops"() -> (w9202:bool)
                              n8715 = local read "VISA Refnum in\nfor Pump"() -> (w9203:refnum<visa-resource-name>)
                              n8716 = case shown="True" w9202 {
                                frame False {
                                }
                                frame True {
                                n8717 = local read "VISA Refnum in\nfor Pump"() -> (w9204:refnum<visa-resource-name>)
                                n8718 = call "HardStopCurrentProcess (SubVI).vi"("VISA Refnum in"=w9204) -> ()  [unwired: 11 in]
                                }
                              }
                              n8719 = call "ProcessCompletionWaiter (SubVI).vi"("VISA Refnum in"=w9203) -> ()  [unwired: 11 in]
                            }
                            frame #7 {
                              # "Keeps the AMF valve after column-1 open and valve after column-2 closed"
                              n8720 = local read "Buffer-B Dispense\nFlow Rate (ul/min)"() -> (w9217:dbl)
                              n8721 = local read "Buffer-B Pumping\nResolution"() -> (w9216:T2)
                              n8722 = local read "VISA Refnum in\nfor Pump"() -> (w9219:refnum<visa-resource-name>)
                              n8723 = local write "Pause Data Collection"(FALSE ("Pause Data Collection")) -> ()
                              n8724 = local write "Valve V1 Open"(TRUE ("Valve V1 Open")) -> ()
                              n8725 = local write "Valve V3 Open"(TRUE ("Valve V3 Open")) -> ()
                              n8726 = local write "Valve V2 Open"(FALSE ("Valve V2 Open")) -> ()
                              n8727 = local write "Valve V4 Open"(TRUE ("Valve V4 Open")) -> ()
                              n8728 = local read "Volume of Syringe"() -> (w9218:dbl)
                              n8729 = call "GoToAbsolutePosition(SubVI).vi"("Absolute Volume Position in Syringe (in ul)"=0.0 ("Volume to be Dispensed"), "Volume of Syringe"=w9218, "Resolution of Pumping"=w9216, "Flow Rate (ul/min)"=w9217, "VISA Refnum in"=w9219) -> ()  [unwired: 6 in, 1 out]
                              n8730 = local write "External Valve \nOpen"(FALSE ("External Valve \nOpen")) -> ()
                              n8731 = local write "Valve V8 Open"(TRUE ("Valve V8 Open")) -> ()
                              n8732 = local write "Valve V6 Open"(TRUE ("Valve V6 Open")) -> ()
                              n8733 = local write "Valve V7 Open"(TRUE ("Valve V7 Open")) -> ()
                              n8734 = local write "Valve V5 Open"(TRUE ("Valve V5 Open")) -> ()
                            }
                            frame #8 {
                              n8735 = local read "Initial Plunger Position"() -> (w9222:dbl)
                              n8736 = local read "Buffer-B Pumping\nResolution"() -> (w9221:T2)
                              n8737 = local read "VISA Refnum in\nfor Pump"() -> (w9223:refnum<visa-resource-name>)
                              n8738 = local read "Volume of Syringe"() -> (w9220:dbl)
                              n8739 = while {
                                tunnel: w9222 -> [w9229]
                                tunnel: w9223 -> [w9228]
                                tunnel: w9221 -> [w9227]
                                tunnel: w9220 -> [w9226]
                                stop <- w9224 stop-if-true
                                n8740 = Wait (ms)(milliseconds to wait=u32 100) -> ()  [unwired: 1 out]
                                n8741 = stacked-sequence {
                                tunnel: w9229 -> [w9235 _]
                                tunnel: w9228 -> [w9234 w9255]
                                tunnel: w9227 -> [w9233 _]
                                tunnel: w9226 -> [w9232 _]
                                tunnel: [_ w9252] -> w9224
                                frame #0 {
                                n8742 = call "AbsolutePlungerPosition (SubVI).vi"("VISA Refnum in"=w9234) -> ("Plunger Position"=w9231:i32)  [unwired: 10 in]
                                n8743 = case shown="\"Standard Pumping\", Default" w9233 {
                                tunnel: w9235 -> [w9240 w9249]
                                tunnel: w9231 -> [w9241 w9248]
                                tunnel: [w9239 w9246] -> w9230
                                tunnel: w9232 -> [w9238 w9247]
                                frame "Standard Pumping", Default {
                                n8744 = Subtract(x=w9240, y=w9241) -> (x-y=w9237:dbl)
                                n8745 = Absolute Value(x=w9237) -> (abs(x)=w9236:dbl)
                                n8746 = Multiply(x=w9236, y=w9238) -> (x*y=w9243:dbl)
                                n8747 = Divide(x=w9243, y=3000.0) -> (x/y=w9239:dbl)
                                }
                                frame "High Resolution Pumping" {
                                n8748 = Subtract(x=w9249, y=w9248) -> (x-y=w9245:dbl)
                                n8749 = Absolute Value(x=w9245) -> (abs(x)=w9244:dbl)
                                n8750 = Multiply(x=w9244, y=w9247) -> (x*y=w9251:dbl)
                                n8751 = Divide(x=w9251, y=24000.0) -> (x/y=w9246:dbl)
                                }
                                }
                                n8752 = local write "Volume being Injected \nin this process"(w9230) -> ()
                                }
                                frame #1 {
                                n8753 = call "LSPOneStatus (SubVI).vi"("VISA Refnum in"=w9255) -> ("read buffer"=w9257:string)  [unwired: 10 in]
                                n8754 = local read "Stopper that ends \nthe main loops"() -> (w9254:bool)
                                n8755 = call <vilib>:"Trim Whitespace.vi"("string"=w9257) -> ("trimmed string"=w9256:string)  [unwired: 1 in]
                                n8756 = Equal?(x=w9256, y="/0`\u0003") -> (x = y?=w9253:bool)
                                n8757 = Or(x=w9253, y=w9254) -> (x .or. y?=w9252:bool)
                                }
                                }
                              }
                            }
                            frame #9 {
                              n8758 = local read "Stopper that ends \nthe main loops"() -> (w9259:bool)
                              n8759 = local write "Pause Data Collection"(TRUE ("Pause Data Collection")) -> ()
                              n8760 = local write "Valve V2 Open"(FALSE ("Valve V2 Open")) -> ()
                              n8761 = Wait (ms)(milliseconds to wait=u32 500) -> ()  [unwired: 1 out]
                              n8762 = local write "Valve V1 Open"(FALSE ("Valve V1 Open")) -> ()
                              n8763 = case shown="True" w9259 {
                                frame False {
                                }
                                frame True {
                                n8764 = local read "VISA Refnum in\nfor Pump"() -> (w9264:refnum<visa-resource-name>)
                                n8765 = call "HardStopCurrentProcess (SubVI).vi"("VISA Refnum in"=w9264) -> ()  [unwired: 11 in]
                                }
                              }
                            }
                            frame #10 {
                              n8766 = local write "Volume being Injected \nin this process"(0.0 ("Volume being Injected \nin this process")) -> ()
                            }
                          }
                        }
                        n8767 = local write "Reminder of the \nVolume to be \nPumped"(w9183) -> ()
                      }
                      frame #1 {
                        n8768 = stacked-sequence {
                          frame #0 {
                            # "Switch to Port-7"
                            # "Port-7 of pump is connected to Buffer-B"
                            n8769 = local read "VISA Refnum in\nfor Pump"() -> (w9267:refnum<visa-resource-name>)
                            n8770 = local read "Port for \nB-Elution"() -> (w9266:string)
                            n8771 = call "PortChanger (SubVI).vi"("Port Number"=w9266, "VISA Refnum in"=w9267) -> ()  [unwired: 10 in]
                          }
                          frame #1 {
                            n8772 = local read "VISA Refnum in\nfor Pump"() -> (w9268:refnum<visa-resource-name>)
                            n8773 = call "ProcessCompletionWaiter (SubVI).vi"("VISA Refnum in"=w9268) -> ()  [unwired: 11 in]
                          }
                          frame #2 {
                            n8774 = local read "Buffer-B PickUp \nFlow Rate (ul/min)"() -> (w9271:dbl)
                            n8775 = local read "Buffer-B Pumping\nResolution"() -> (w9270:T2)
                            n8776 = local read "VISA Refnum in\nfor Pump"() -> (w9273:refnum<visa-resource-name>)
                            n8777 = local read "Reminder of the \nVolume to be \nPumped"() -> (w9269:dbl)
                            n8778 = local read "Volume of Syringe"() -> (w9272:dbl)
                            n8779 = call "RPickUp(SubVI).vi"("Volume to be picked up"=w9269, "Volume of Syringe"=w9272, "Resolution of PickUP"=w9270, "PickUp Flow Rate (ul/min)"=w9271, "VISA Refnum in"=w9273) -> ()  [unwired: 6 in, 1 out]
                          }
                          frame #3 {
                            n8780 = local read "Stopper that ends \nthe main loops"() -> (w9274:bool)
                            n8781 = local read "VISA Refnum in\nfor Pump"() -> (w9275:refnum<visa-resource-name>)
                            n8782 = case shown="True" w9274 {
                              frame False {
                              }
                              frame True {
                                n8783 = local read "VISA Refnum in\nfor Pump"() -> (w9276:refnum<visa-resource-name>)
                                n8784 = call "HardStopCurrentProcess (SubVI).vi"("VISA Refnum in"=w9276) -> ()  [unwired: 11 in]
                              }
                            }
                            n8785 = call "ProcessCompletionWaiter (SubVI).vi"("VISA Refnum in"=w9275) -> ()  [unwired: 11 in]
                          }
                          frame #4 {
                            # "Reads the initial Plunger Position for computing the volume dispensed"
                            n8786 = local read "VISA Refnum in\nfor Pump"() -> (w9278:refnum<visa-resource-name>)
                            n8787 = call "AbsolutePlungerPosition (SubVI).vi"("VISA Refnum in"=w9278) -> ("Plunger Position"=w9277:i32)  [unwired: 10 in]
                            n8788 = local write "Initial Plunger Position"(w9277) -> ()
                          }
                          frame #5 {
                            # "Switch to Port-2"
                            # "Port-2 of the pump is conncted to column-1 of chip"
                            n8789 = local read "VISA Refnum in\nfor Pump"() -> (w9280:refnum<visa-resource-name>)
                            n8790 = call "PortChanger (SubVI).vi"("Port Number"="8", "VISA Refnum in"=w9280) -> ()  [unwired: 10 in]
                          }
                          frame #6 {
                            n8791 = local read "Stopper that ends \nthe main loops"() -> (w9281:bool)
                            n8792 = local read "VISA Refnum in\nfor Pump"() -> (w9282:refnum<visa-resource-name>)
                            n8793 = case shown="True" w9281 {
                              frame False {
                              }
                              frame True {
                                n8794 = local read "VISA Refnum in\nfor Pump"() -> (w9283:refnum<visa-resource-name>)
                                n8795 = call "HardStopCurrentProcess (SubVI).vi"("VISA Refnum in"=w9283) -> ()  [unwired: 11 in]
                              }
                            }
                            n8796 = call "ProcessCompletionWaiter (SubVI).vi"("VISA Refnum in"=w9282) -> ()  [unwired: 11 in]
                          }
                          frame #7 {
                            # "Keeps the AMF valve after column-1 open and valve after column-2 closed"
                            n8797 = local read "Buffer-B Dispense\nFlow Rate (ul/min)"() -> (w9296:dbl)
                            n8798 = local read "Buffer-B Pumping\nResolution"() -> (w9295:T2)
                            n8799 = local read "VISA Refnum in\nfor Pump"() -> (w9298:refnum<visa-resource-name>)
                            n8800 = local write "Pause Data Collection"(FALSE ("Pause Data Collection")) -> ()
                            n8801 = local write "Valve V1 Open"(TRUE ("Valve V1 Open")) -> ()
                            n8802 = local write "Valve V3 Open"(TRUE ("Valve V3 Open")) -> ()
                            n8803 = local write "Valve V2 Open"(FALSE ("Valve V2 Open")) -> ()
                            n8804 = local write "Valve V4 Open"(TRUE ("Valve V4 Open")) -> ()
                            n8805 = local read "Volume of Syringe"() -> (w9297:dbl)
                            n8806 = call "GoToAbsolutePosition(SubVI).vi"("Absolute Volume Position in Syringe (in ul)"=0.0 ("Volume to be Dispensed"), "Volume of Syringe"=w9297, "Resolution of Pumping"=w9295, "Flow Rate (ul/min)"=w9296, "VISA Refnum in"=w9298) -> ()  [unwired: 6 in, 1 out]
                            n8807 = local write "External Valve \nOpen"(FALSE ("External Valve \nOpen")) -> ()
                            n8808 = local write "Valve V8 Open"(TRUE ("Valve V8 Open")) -> ()
                            n8809 = local write "Valve V6 Open"(TRUE ("Valve V6 Open")) -> ()
                            n8810 = local write "Valve V7 Open"(TRUE ("Valve V7 Open")) -> ()
                            n8811 = local write "Valve V5 Open"(TRUE ("Valve V5 Open")) -> ()
                          }
                          frame #8 {
                            n8812 = local read "Initial Plunger Position"() -> (w9301:dbl)
                            n8813 = local read "Buffer-B Pumping\nResolution"() -> (w9300:T2)
                            n8814 = local read "VISA Refnum in\nfor Pump"() -> (w9302:refnum<visa-resource-name>)
                            n8815 = local read "Volume of Syringe"() -> (w9299:dbl)
                            n8816 = while {
                              tunnel: w9301 -> [w9308]
                              tunnel: w9302 -> [w9307]
                              tunnel: w9300 -> [w9306]
                              tunnel: w9299 -> [w9305]
                              stop <- w9303 stop-if-true
                              n8817 = Wait (ms)(milliseconds to wait=u32 100) -> ()  [unwired: 1 out]
                              n8818 = stacked-sequence {
                                tunnel: w9308 -> [w9314 _]
                                tunnel: w9307 -> [w9313 w9334]
                                tunnel: w9306 -> [w9312 _]
                                tunnel: w9305 -> [w9311 _]
                                tunnel: [_ w9331] -> w9303
                                frame #0 {
                                n8819 = call "AbsolutePlungerPosition (SubVI).vi"("VISA Refnum in"=w9313) -> ("Plunger Position"=w9310:i32)  [unwired: 10 in]
                                n8820 = case shown="\"Standard Pumping\", Default" w9312 {
                                tunnel: w9314 -> [w9319 w9328]
                                tunnel: w9310 -> [w9320 w9327]
                                tunnel: [w9318 w9325] -> w9309
                                tunnel: w9311 -> [w9317 w9326]
                                frame "Standard Pumping", Default {
                                n8821 = Subtract(x=w9319, y=w9320) -> (x-y=w9316:dbl)
                                n8822 = Absolute Value(x=w9316) -> (abs(x)=w9315:dbl)
                                n8823 = Multiply(x=w9315, y=w9317) -> (x*y=w9322:dbl)
                                n8824 = Divide(x=w9322, y=3000.0) -> (x/y=w9318:dbl)
                                }
                                frame "High Resolution Pumping" {
                                n8825 = Subtract(x=w9328, y=w9327) -> (x-y=w9324:dbl)
                                n8826 = Absolute Value(x=w9324) -> (abs(x)=w9323:dbl)
                                n8827 = Multiply(x=w9323, y=w9326) -> (x*y=w9330:dbl)
                                n8828 = Divide(x=w9330, y=24000.0) -> (x/y=w9325:dbl)
                                }
                                }
                                n8829 = local write "Volume being Injected \nin this process"(w9309) -> ()
                                }
                                frame #1 {
                                n8830 = call "LSPOneStatus (SubVI).vi"("VISA Refnum in"=w9334) -> ("read buffer"=w9336:string)  [unwired: 10 in]
                                n8831 = local read "Stopper that ends \nthe main loops"() -> (w9333:bool)
                                n8832 = call <vilib>:"Trim Whitespace.vi"("string"=w9336) -> ("trimmed string"=w9335:string)  [unwired: 1 in]
                                n8833 = Equal?(x=w9335, y="/0`\u0003") -> (x = y?=w9332:bool)
                                n8834 = Or(x=w9332, y=w9333) -> (x .or. y?=w9331:bool)
                                }
                              }
                            }
                          }
                          frame #9 {
                            n8835 = local read "Stopper that ends \nthe main loops"() -> (w9338:bool)
                            n8836 = local write "Pause Data Collection"(TRUE ("Pause Data Collection")) -> ()
                            n8837 = local write "Valve V2 Open"(FALSE ("Valve V2 Open")) -> ()
                            n8838 = local write "Start the Process"(FALSE) -> ()
                            n8839 = Wait (ms)(milliseconds to wait=u32 500) -> ()  [unwired: 1 out]
                            n8840 = local write "Valve V1 Open"(FALSE ("Valve V1 Open")) -> ()
                            n8841 = case shown="True" w9338 {
                              frame False {
                              }
                              frame True {
                                n8842 = local read "VISA Refnum in\nfor Pump"() -> (w9344:refnum<visa-resource-name>)
                                n8843 = call "HardStopCurrentProcess (SubVI).vi"("VISA Refnum in"=w9344) -> ()  [unwired: 11 in]
                              }
                            }
                          }
                          frame #10 {
                            n8844 = local write "Volume being Injected \nin this process"(0.0 ("Volume being Injected \nin this process")) -> ()
                          }
                        }
                      }
                    }
                  }
                }
              }
              frame True {
                n8845 = local write "Pause Data Collection"(FALSE ("Pause Data Collection")) -> ()
              }
            }
          }
          frame "Inject Buffer C2, Column 2 with 4 SOD Valves" {
            n8846 = local read "Stopper that ends \nthe main loops"() -> (w9347:bool)
            n8847 = case shown="False" w9347 {
              frame False {
                n8848 = local read "Start the Process"() -> (w9348:bool)
                n8849 = case shown="True" w9348 {
                  frame False {
                    n8850 = local read "Stopper that ends \nthe main loops"() -> (w9350:bool)
                    n8851 = local read "Start the Process"() -> (w9349:bool)
                    n8852 = Or(x=w9350, y=w9349) -> (x .or. y?=w9351:bool)
                    n8853 = case shown="False" w9351 {
                      frame False {
                        n8854 = while {
                          stop <- w9354 stop-if-true
                          n8855 = local read "Stop for End of \nExperiment \nand Data Writing"() -> (w9353:bool)
                          n8856 = local read "Stopper that ends \nthe main loops"() -> (w9356:bool)
                          n8857 = local read "Start the Process"() -> (w9355:bool)
                          n8858 = Wait (ms)(milliseconds to wait=u32 10) -> ()  [unwired: 1 out]
                          n8859 = Or(x=w9356, y=w9355) -> (x .or. y?=w9354:bool)
                          n8860 = local write "Stopper that ends \nthe main loops"(w9353) -> ()
                        }
                        n8861 = One Button Dialog(message="Please Select the Process and Press 'Start the Process' Button") -> ()  [unwired: 1 in, 1 out]
                      }
                      frame True {
                      }
                    }
                  }
                  frame True {
                    n8862 = stacked-sequence {
                      frame #0 {
                        n8863 = local read "Apparent Volume\nof Syringe"() -> (w9360:dbl)
                        n8864 = local read "Buffer-C2 Volume \nto be Pumped"() -> (w9361:dbl)
                        n8865 = Quotient & Remainder(x=w9361, y=w9360) -> (x-y*floor(x/y)=w9358:dbl, floor(x/y)=w9359:dbl)
                        n8866 = for {
                          N: w9359 -> [_]
                          n8867 = stacked-sequence {
                            frame #0 {
                              # "Switch to Port-5/8"
                              # "Port-5/8 of pump is connected to Buffer-C/Buffer-A"
                              n8868 = local read "VISA Refnum in\nfor Pump"() -> (w9363:refnum<visa-resource-name>)
                              n8869 = local read "Port for \nC2-Elution"() -> (w9362:string)
                              n8870 = call "PortChanger (SubVI).vi"("Port Number"=w9362, "VISA Refnum in"=w9363) -> ()  [unwired: 10 in]
                            }
                            frame #1 {
                              n8871 = local read "VISA Refnum in\nfor Pump"() -> (w9364:refnum<visa-resource-name>)
                              n8872 = call "ProcessCompletionWaiter (SubVI).vi"("VISA Refnum in"=w9364) -> ()  [unwired: 11 in]
                            }
                            frame #2 {
                              n8873 = local read "Buffer-C2 PickUp \nFlow Rate (ul/min)"() -> (w9367:dbl)
                              n8874 = local read "Buffer-C2 Pumping\nResolution"() -> (w9366:T2)
                              n8875 = local read "VISA Refnum in\nfor Pump"() -> (w9369:refnum<visa-resource-name>)
                              n8876 = local read "Apparent Volume\nof Syringe"() -> (w9365:dbl)
                              n8877 = local read "Volume of Syringe"() -> (w9368:dbl)
                              n8878 = call "RPickUp(SubVI).vi"("Volume to be picked up"=w9365, "Volume of Syringe"=w9368, "Resolution of PickUP"=w9366, "PickUp Flow Rate (ul/min)"=w9367, "VISA Refnum in"=w9369) -> ()  [unwired: 6 in, 1 out]
                            }
                            frame #3 {
                              n8879 = local read "Stopper that ends \nthe main loops"() -> (w9370:bool)
                              n8880 = local read "VISA Refnum in\nfor Pump"() -> (w9371:refnum<visa-resource-name>)
                              n8881 = case shown="True" w9370 {
                                frame False {
                                }
                                frame True {
                                n8882 = local read "VISA Refnum in\nfor Pump"() -> (w9372:refnum<visa-resource-name>)
                                n8883 = call "HardStopCurrentProcess (SubVI).vi"("VISA Refnum in"=w9372) -> ()  [unwired: 11 in]
                                }
                              }
                              n8884 = call "ProcessCompletionWaiter (SubVI).vi"("VISA Refnum in"=w9371) -> ()  [unwired: 11 in]
                            }
                            frame #4 {
                              # "Reads the initial Plunger Position for computing the volume dispensed"
                              n8885 = local read "VISA Refnum in\nfor Pump"() -> (w9374:refnum<visa-resource-name>)
                              n8886 = call "AbsolutePlungerPosition (SubVI).vi"("VISA Refnum in"=w9374) -> ("Plunger Position"=w9373:i32)  [unwired: 10 in]
                              n8887 = local write "Initial Plunger Position"(w9373) -> ()
                            }
                            frame #5 {
                              # "Switch to Port-10"
                              # "Port-10 of the pump is conncted to column-2 of chip"
                              n8888 = local read "VISA Refnum in\nfor Pump"() -> (w9376:refnum<visa-resource-name>)
                              n8889 = call "PortChanger (SubVI).vi"("Port Number"="10", "VISA Refnum in"=w9376) -> ()  [unwired: 10 in]
                            }
                            frame #6 {
                              n8890 = local read "Stopper that ends \nthe main loops"() -> (w9377:bool)
                              n8891 = local read "VISA Refnum in\nfor Pump"() -> (w9378:refnum<visa-resource-name>)
                              n8892 = case shown="True" w9377 {
                                frame False {
                                }
                                frame True {
                                n8893 = local read "VISA Refnum in\nfor Pump"() -> (w9379:refnum<visa-resource-name>)
                                n8894 = call "HardStopCurrentProcess (SubVI).vi"("VISA Refnum in"=w9379) -> ()  [unwired: 11 in]
                                }
                              }
                              n8895 = call "ProcessCompletionWaiter (SubVI).vi"("VISA Refnum in"=w9378) -> ()  [unwired: 11 in]
                            }
                            frame #7 {
                              # "Keeps the AMF valve after column-1 closed and valve after column-2 open"
                              n8896 = local read "Buffer-C2 Dispense\nFlow Rate (ul/min)"() -> (w9392:dbl)
                              n8897 = local read "Buffer-C2 Pumping\nResolution"() -> (w9391:T2)
                              n8898 = local read "VISA Refnum in\nfor Pump"() -> (w9394:refnum<visa-resource-name>)
                              n8899 = local write "Pause Data Collection"(FALSE ("Pause Data Collection")) -> ()
                              n8900 = local write "Valve V1 Open"(FALSE ("Valve V1 Open")) -> ()
                              n8901 = local write "Valve V3 Open"(TRUE ("Valve V3 Open")) -> ()
                              n8902 = local write "Valve V2 Open"(FALSE ("Valve V2 Open")) -> ()
                              n8903 = local write "Valve V4 Open"(TRUE ("Valve V4 Open")) -> ()
                              n8904 = local read "Volume of Syringe"() -> (w9393:dbl)
                              n8905 = call "GoToAbsolutePosition(SubVI).vi"("Absolute Volume Position in Syringe (in ul)"=0.0 ("Volume to be Dispensed"), "Volume of Syringe"=w9393, "Resolution of Pumping"=w9391, "Flow Rate (ul/min)"=w9392, "VISA Refnum in"=w9394) -> ()  [unwired: 6 in, 1 out]
                              n8906 = local write "External Valve \nOpen"(FALSE ("External Valve \nOpen")) -> ()
                              n8907 = local write "Valve V8 Open"(FALSE ("Valve V8 Open")) -> ()
                              n8908 = local write "Valve V7 Open"(TRUE ("Valve V7 Open")) -> ()
                              n8909 = local write "Valve V6 Open"(FALSE ("Valve V6 Open")) -> ()
                              n8910 = local write "Valve V5 Open"(TRUE ("Valve V5 Open")) -> ()
                            }
                            frame #8 {
                              n8911 = local read "Initial Plunger Position"() -> (w9397:dbl)
                              n8912 = local read "Buffer-C2 Pumping\nResolution"() -> (w9396:T2)
                              n8913 = local read "VISA Refnum in\nfor Pump"() -> (w9398:refnum<visa-resource-name>)
                              n8914 = local read "Volume of Syringe"() -> (w9395:dbl)
                              n8915 = while {
                                tunnel: w9397 -> [w9404]
                                tunnel: w9398 -> [w9403]
                                tunnel: w9396 -> [w9402]
                                tunnel: w9395 -> [w9401]
                                stop <- w9399 stop-if-true
                                n8916 = Wait (ms)(milliseconds to wait=u32 100) -> ()  [unwired: 1 out]
                                n8917 = stacked-sequence {
                                tunnel: w9404 -> [w9410 _]
                                tunnel: w9403 -> [w9409 w9430]
                                tunnel: w9402 -> [w9408 _]
                                tunnel: w9401 -> [w9407 _]
                                tunnel: [_ w9427] -> w9399
                                frame #0 {
                                n8918 = call "AbsolutePlungerPosition (SubVI).vi"("VISA Refnum in"=w9409) -> ("Plunger Position"=w9406:i32)  [unwired: 10 in]
                                n8919 = case shown="\"Standard Pumping\", Default" w9408 {
                                tunnel: w9410 -> [w9415 w9424]
                                tunnel: w9406 -> [w9416 w9423]
                                tunnel: [w9414 w9421] -> w9405
                                tunnel: w9407 -> [w9413 w9422]
                                frame "Standard Pumping", Default {
                                n8920 = Subtract(x=w9415, y=w9416) -> (x-y=w9412:dbl)
                                n8921 = Absolute Value(x=w9412) -> (abs(x)=w9411:dbl)
                                n8922 = Multiply(x=w9411, y=w9413) -> (x*y=w9418:dbl)
                                n8923 = Divide(x=w9418, y=3000.0) -> (x/y=w9414:dbl)
                                }
                                frame "High Resolution Pumping" {
                                n8924 = Subtract(x=w9424, y=w9423) -> (x-y=w9420:dbl)
                                n8925 = Absolute Value(x=w9420) -> (abs(x)=w9419:dbl)
                                n8926 = Multiply(x=w9419, y=w9422) -> (x*y=w9426:dbl)
                                n8927 = Divide(x=w9426, y=24000.0) -> (x/y=w9421:dbl)
                                }
                                }
                                n8928 = local write "Volume being Injected \nin this process"(w9405) -> ()
                                }
                                frame #1 {
                                n8929 = local read "Stop for End of \nExperiment \nand Data Writing"() -> (w9429:bool)
                                n8930 = call "LSPOneStatus (SubVI).vi"("VISA Refnum in"=w9430) -> ("read buffer"=w9432:string)  [unwired: 10 in]
                                n8931 = call <vilib>:"Trim Whitespace.vi"("string"=w9432) -> ("trimmed string"=w9431:string)  [unwired: 1 in]
                                n8932 = Equal?(x=w9431, y="/0`\u0003") -> (x = y?=w9428:bool)
                                n8933 = Or(x=w9428, y=w9429) -> (x .or. y?=w9427:bool)
                                }
                                }
                              }
                            }
                            frame #9 {
                              n8934 = local read "Stop for End of \nExperiment \nand Data Writing"() -> (w9434:bool)
                              n8935 = local write "Pause Data Collection"(TRUE ("Pause Data Collection")) -> ()
                              n8936 = local write "Valve V2 Open"(FALSE ("Valve V2 Open")) -> ()
                              n8937 = local write "Valve V1 Open"(FALSE ("Valve V1 Open")) -> ()
                              n8938 = local write "Valve V3 Open"(FALSE ("Valve V3 Open")) -> ()
                              n8939 = local write "Valve V4 Open"(FALSE ("Valve V4 Open")) -> ()
                              n8940 = Wait (ms)(milliseconds to wait=u32 500) -> ()  [unwired: 1 out]
                              n8941 = case shown="True" w9434 {
                                frame False {
                                }
                                frame True {
                                n8942 = local read "VISA Refnum in\nfor Pump"() -> (w9444:refnum<visa-resource-name>)
                                n8943 = call "HardStopCurrentProcess (SubVI).vi"("VISA Refnum in"=w9444) -> ()  [unwired: 11 in]
                                }
                              }
                              n8944 = local write "Valve V6 Open"(FALSE ("Valve V6 Open")) -> ()
                              n8945 = local write "Valve V5 Open"(FALSE ("Valve V5 Open")) -> ()
                              n8946 = local write "Valve V7 Open"(FALSE ("Valve V7 Open")) -> ()
                            }
                            frame #10 {
                              n8947 = local write "Volume being Injected \nin this process"(0.0 ("Volume being Injected \nin this process")) -> ()
                            }
                          }
                        }
                        n8948 = local write "Reminder of the \nVolume to be \nPumped"(w9358) -> ()
                      }
                      frame #1 {
                        n8949 = stacked-sequence {
                          frame #0 {
                            # "Switch to Port-5/8"
                            # "Port-5/8 of pump is connected to Buffer-C/Buffer-A"
                            n8950 = local read "VISA Refnum in\nfor Pump"() -> (w9447:refnum<visa-resource-name>)
                            n8951 = local read "Port for \nC2-Elution"() -> (w9446:string)
                            n8952 = call "PortChanger (SubVI).vi"("Port Number"=w9446, "VISA Refnum in"=w9447) -> ()  [unwired: 10 in]
                          }
                          frame #1 {
                            n8953 = local read "VISA Refnum in\nfor Pump"() -> (w9448:refnum<visa-resource-name>)
                            n8954 = call "ProcessCompletionWaiter (SubVI).vi"("VISA Refnum in"=w9448) -> ()  [unwired: 11 in]
                          }
                          frame #2 {
                            n8955 = local read "Buffer-C2 PickUp \nFlow Rate (ul/min)"() -> (w9451:dbl)
                            n8956 = local read "Buffer-C2 Pumping\nResolution"() -> (w9450:T2)
                            n8957 = local read "VISA Refnum in\nfor Pump"() -> (w9453:refnum<visa-resource-name>)
                            n8958 = local read "Reminder of the \nVolume to be \nPumped"() -> (w9449:dbl)
                            n8959 = local read "Volume of Syringe"() -> (w9452:dbl)
                            n8960 = call "RPickUp(SubVI).vi"("Volume to be picked up"=w9449, "Volume of Syringe"=w9452, "Resolution of PickUP"=w9450, "PickUp Flow Rate (ul/min)"=w9451, "VISA Refnum in"=w9453) -> ()  [unwired: 6 in, 1 out]
